vi "DowngradeFatalErrorToDWarn.vi"(7 "DWarnInternal? (false)":bool, 8 "error in":errorcluster, 11 "String to prepend on downgrade":string) -> (0 "error out":errorcluster)   [LabVIEW 2020, in "NI_XNodeSupport.lvlib"]
uses:
  <vilib>/XNodeSupport/NI_XNodeSupport.lvlib
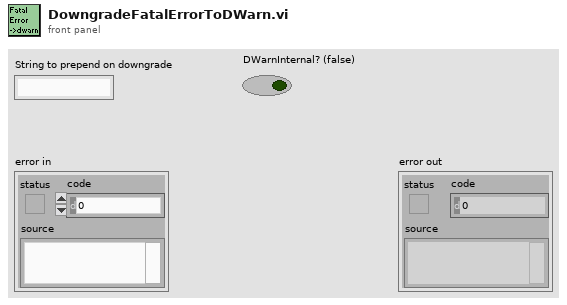
[diagram p1: front panel]
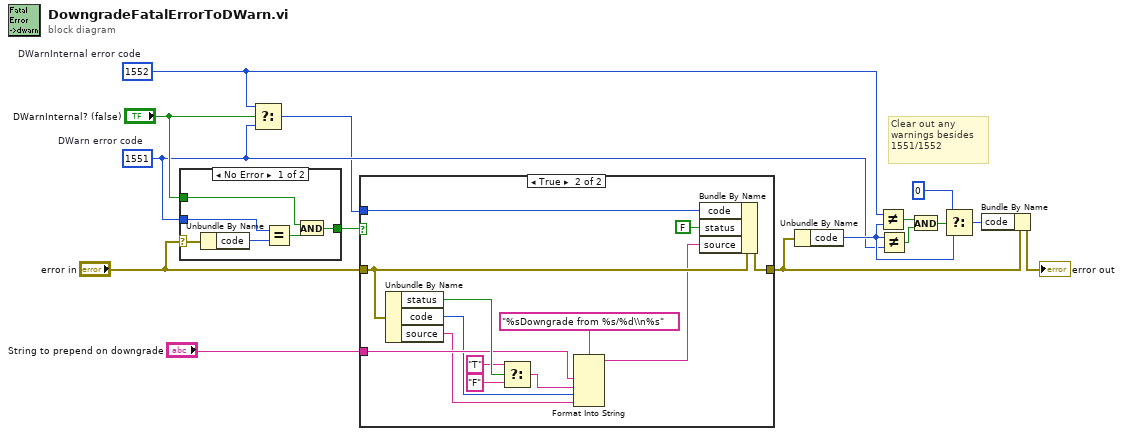
[diagram p0: block diagram]
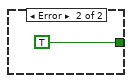
[diagram p2: hidden frame]
diagram:
  w3 = 1551  # DWarn error code
  w4 = 1552  # DWarnInternal error code
  # "Clear out any warnings besides 1551/1552"
  n1 = case shown="No Error" "error in" {
    selector: "error in" -> [w21 _]
    tunnel: "DWarnInternal? (false)" -> [w19 _]
    tunnel: w3 -> [w17 _]
    tunnel: [w16 TRUE] -> w6
    frame No Error {
      n2 = Unbundle By Name(w21) -> ("code"=w18:i32)
      n3 = Equal?(x=w17, y=w18) -> (x = y?=w20:bool)
      n4 = And(x=w19, y=w20) -> (x .and. y?=w16:bool)
    }
    frame Error {
    }
  }
  n5 = Select(t=w4, s="DWarnInternal? (false)", f=w3) -> (s? t:f=w2:i32)
  n6 = case shown="True" w6 {
    tunnel: w2 -> [_ w34]
    tunnel: "error in" -> [w23 w36]
    tunnel: [w23 w35] -> w13
    tunnel: "String to prepend on downgrade" -> [_ w27]
    frame False {
    }
    frame True {
      n7 = Unbundle By Name(w36) -> ("status"=w31:bool, "code"=w26:i32, "source"=w24:string)
      n8 = Select(t="T" ("String to prepend on downgrade"), s=w31, f="F" ("String to prepend on downgrade")) -> (s? t:f=w28:string)
      n9 = Format Into String(format string="%sDowngrade from %s/%d\\n%s", w27, w28, w26, w24) -> (resulting string=w25:string)  [unwired: 2 in, 1 out]
      n10 = Bundle By Name(cluster=w36, "code"=w34, "status"=FALSE, "source"=w25) -> (w35:errorcluster)
    }
  }
  n11 = Unbundle By Name(w13) -> ("code"=w11:i32)
  n12 = Not Equal?(x=w4, y=w11) -> (x != y?=w8:bool)
  n13 = Not Equal?(x=w11, y=w3) -> (x != y?=w9:bool)
  n14 = And(x=w8, y=w9) -> (x .and. y?=w10:bool)
  n15 = Select(t=0, s=w10, f=w11) -> (s? t:f=w7:i32)
  n16 = Bundle By Name(cluster=w13, "code"=w7) -> (→"error out":errorcluster)
